vi "Force Measurement.vi"() -> ()   [LabVIEW 2017]
uses:
  <vilib>/Analysis/baseanly.llb/Mean (DBL).vi
  Documents/WT-Control/NU-LabVIEW/Globals/mainWTControl.vi
  <vilib>/Analysis/NI_AALBase.lvlib
panel:
  out "Temp 2":dbl(graph)
  out "Fx":dbl(graph)
  out "Start time":timestamp
  out "concatenated string":string
  in  "Stop Button":bool
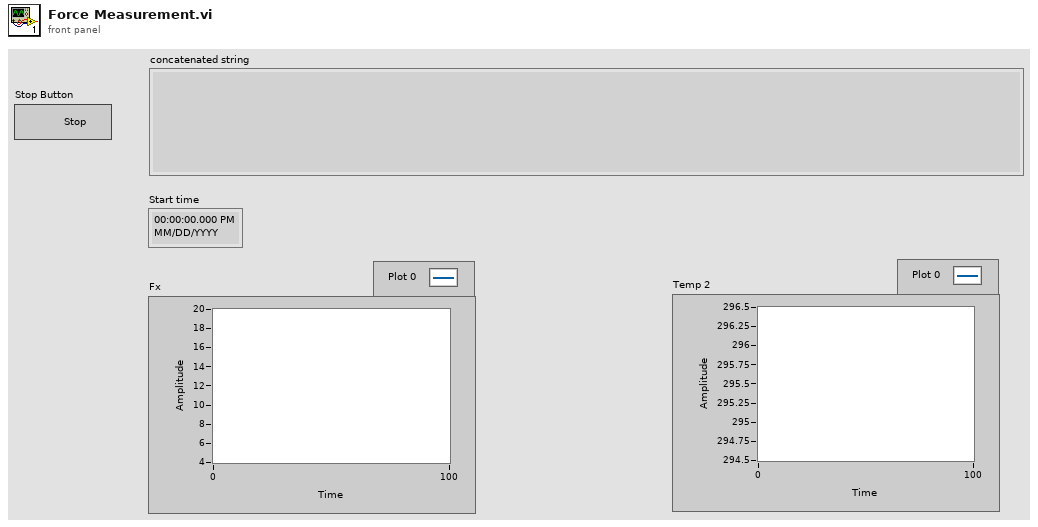
[diagram p1: front panel]
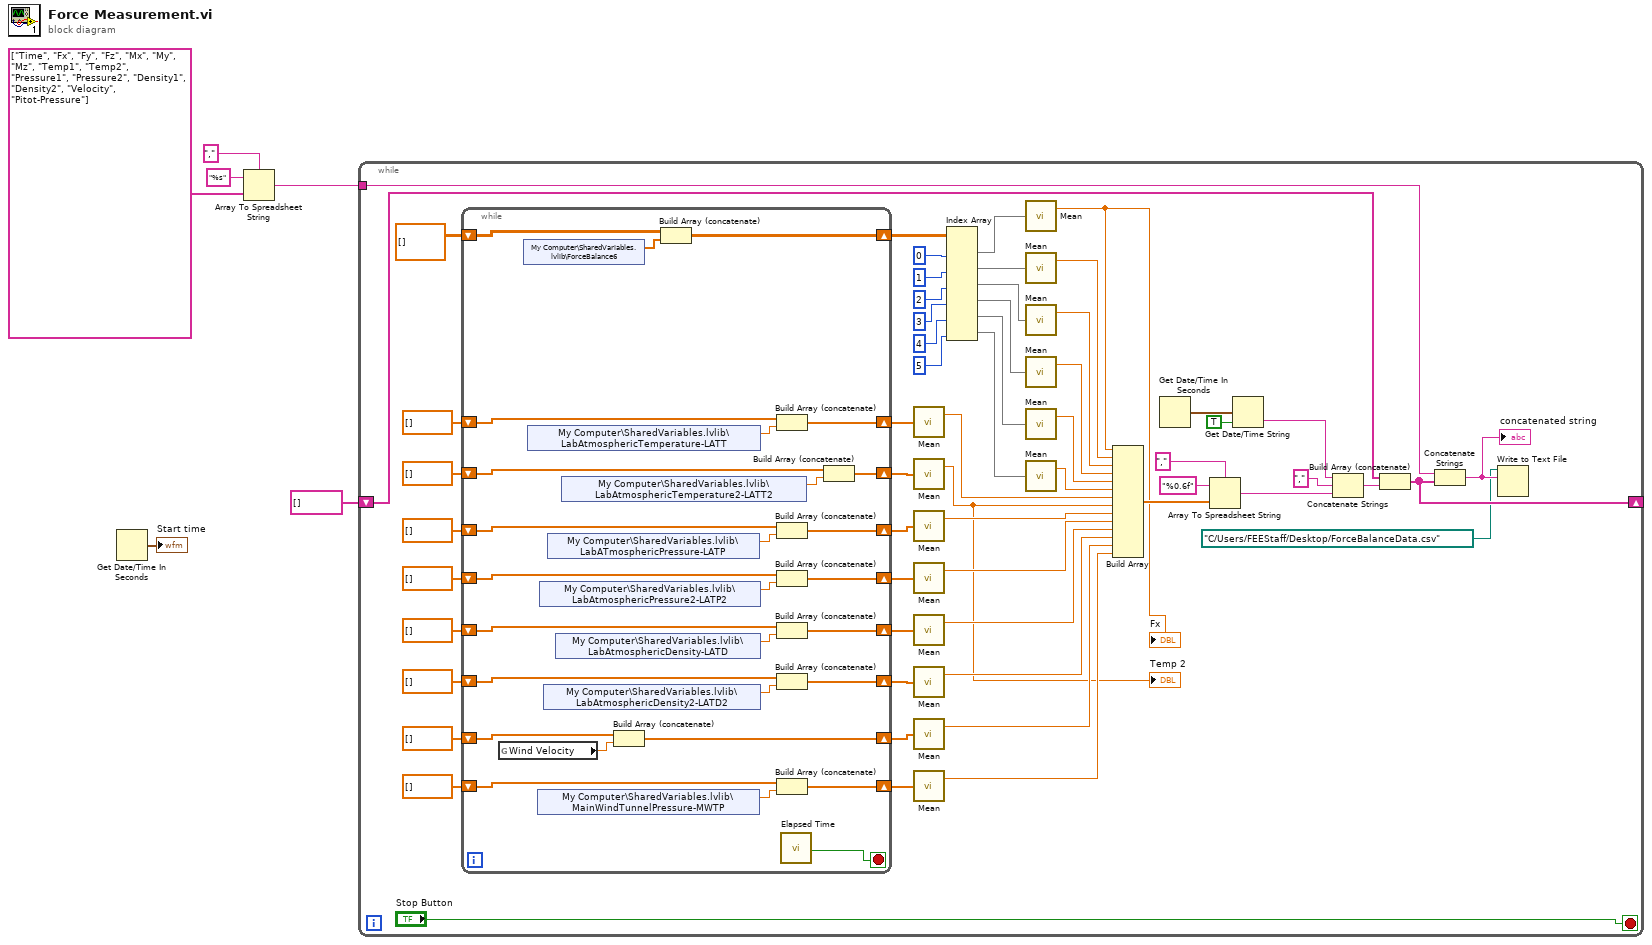
[diagram p0: block diagram]
diagram:
  n1 = Get Date/Time In Seconds() -> (seconds since 1Jan1904=→"Start time":timestamp)
  n2 = Array To Spreadsheet String(delimiter (Tab)=",", array=string[] ["Time", "Fx", "Fy", "Fz", "Mx", "My", "Mz", "Temp1", "Temp2", "Pressure1", "Pressure2", "Density1", "Density2", "Velocity", "Pitot-Pressure"], 3:"%s" ("delimiter (Tab)")) -> (spreadsheet string=w2:string)
  n3 = while {
    shift-right: [w54] -> _
    shift-left: string[] [] -> [w56]
    tunnel: w2 -> [w55]
    stop <- "Stop Button" stop-if-true
    n4 = while {
      shift-right: [w92] -> w52
      shift-left: dbl[][] [] -> [w91]
      shift-right: [w88] -> w38
      shift-left: dbl[] [] -> [w87]
      shift-right: [w73] -> w31
      shift-left: dbl[] [] -> [w66]
      shift-right: [w75] -> w33
      shift-left: dbl[] [] -> [w68]
      shift-right: [w74] -> w32
      shift-left: dbl[] [] -> [w67]
      shift-right: [w76] -> w34
      shift-left: dbl[] [] -> [w69]
      shift-right: [w77] -> w35
      shift-left: dbl[] [] -> [w70]
      shift-right: [w78] -> w36
      shift-left: dbl[] [] -> [w71]
      shift-right: [w85] -> w37
      shift-left: dbl[] [] -> [w72]
      stop <- w90 stop-if-true
      n5 = global read "mainWTControl.vi" "Wind Velocity"() -> (w80:dbl)
      n6 = shared-variable "My Computer\\SharedVariables.lvlib\\ForceBalance6"() -> (w93:dbl[])  [unwired: 1 in, 1 out]
      n7 = shared-variable "My Computer\\SharedVariables.lvlib\\LabAtmosphericTemperature-LATT"() -> (w89:dbl)  [unwired: 1 in, 1 out]
      n8 = shared-variable "My Computer\\SharedVariables.lvlib\\MainWindTunnelPressure-MWTP"() -> (w79:dbl)  [unwired: 1 in, 1 out]
      n9 = shared-variable "My Computer\\SharedVariables.lvlib\\LabAtmosphericPressure2-LATP2"() -> (w83:dbl)  [unwired: 1 in, 1 out]
      n10 = shared-variable "My Computer\\SharedVariables.lvlib\\LabAtmosphericDensity2-LATD2"() -> (w81:dbl)  [unwired: 1 in, 1 out]
      n11 = shared-variable "My Computer\\SharedVariables.lvlib\\LabATmosphericPressure-LATP"() -> (w84:dbl)  [unwired: 1 in, 1 out]
      n12 = shared-variable "My Computer\\SharedVariables.lvlib\\LabAtmosphericDensity-LATD"() -> (w82:dbl)  [unwired: 1 in, 1 out]
      n13 = shared-variable "My Computer\\SharedVariables.lvlib\\LabAtmosphericTemperature2-LATT2"() -> (w86:dbl)  [unwired: 1 in, 1 out]
      n14 = Build Array (concatenate)(w67, w80) -> (w74:dbl[])
      n15 = Build Array (concatenate)(w91, w93) -> (w92:dbl[][])
      n16 = Build Array (concatenate)(w87, w89) -> (w88:dbl[])
      n17 = Build Array (concatenate)(w71, w84) -> (w78:dbl[])
      n18 = Build Array (concatenate)(w70, w83) -> (w77:dbl[])
      n19 = Build Array (concatenate)(w69, w82) -> (w76:dbl[])
      n20 = Build Array (concatenate)(w68, w81) -> (w75:dbl[])
      n21 = Build Array (concatenate)(w66, w79) -> (w73:dbl[])
      n22 = call "Elapsed Time"() -> ("Time has Elapsed"=w90:bool)  [unwired: 12 in, 7 out]
      n23 = Build Array (concatenate)(w72, w86) -> (w85:dbl[])
    }
    n24 = call-poly <vilib>:"Mean.vi"("X"=w38) -> ("mean"=w17:dbl)  [unwired: 1 out]
    n25 = call-poly <vilib>:"Mean.vi"("X"=w37) -> ("mean"=w16:dbl)  [unwired: 1 out]
    "Temp 2" <- w16
    n26 = call-poly <vilib>:"Mean.vi"("X"=w36) -> ("mean"=w25:dbl)  [unwired: 1 out]
    n27 = call-poly <vilib>:"Mean.vi"("X"=w35) -> ("mean"=w24:dbl)  [unwired: 1 out]
    n28 = call-poly <vilib>:"Mean.vi"("X"=w34) -> ("mean"=w23:dbl)  [unwired: 1 out]
    n29 = call-poly <vilib>:"Mean.vi"("X"=w33) -> ("mean"=w22:dbl)  [unwired: 1 out]
    n30 = call-poly <vilib>:"Mean.vi"("X"=w32) -> ("mean"=w21:dbl)  [unwired: 1 out]
    n31 = call-poly <vilib>:"Mean.vi"("X"=w31) -> ("mean"=w20:dbl)  [unwired: 1 out]
    n32 = Index Array(array=w52, index (col) #1=0 ("disabled index (col)"), index (col) #2=1 ("index (col)"), index (col) #3=2 ("index (col)"), index (col) #4=3 ("index (col)"), index (col) #5=4 ("index (col)"), index (col) #6=5 ("index (col)")) -> (element #1=w45:dbl[], element #2=w44:dbl[], element #3=w43:dbl[], element #4=w42:dbl[], element #5=w41:dbl[], element #6=w40:dbl[])  [unwired: 6 in]
    n33 = call-poly <vilib>:"Mean.vi"("X"=w45) -> ("mean"=w7:dbl)  [unwired: 1 out]
    "Fx" <- w7
    n34 = call-poly <vilib>:"Mean.vi"("X"=w44) -> ("mean"=w30:dbl)  [unwired: 1 out]
    n35 = call-poly <vilib>:"Mean.vi"("X"=w43) -> ("mean"=w29:dbl)  [unwired: 1 out]
    n36 = call-poly <vilib>:"Mean.vi"("X"=w42) -> ("mean"=w28:dbl)  [unwired: 1 out]
    n37 = call-poly <vilib>:"Mean.vi"("X"=w41) -> ("mean"=w27:dbl)  [unwired: 1 out]
    n38 = call-poly <vilib>:"Mean.vi"("X"=w40) -> ("mean"=w26:dbl)  [unwired: 1 out]
    n39 = Build Array(w7, w30, w29, w28, w27, w26, w17, w16, w25, w24, w23, w22, w21, w20) -> (w39:dbl[])
    n40 = Get Date/Time In Seconds() -> (seconds since 1Jan1904=w62:timestamp)
    n41 = Array To Spreadsheet String(delimiter (Tab)=",", array=w39, 3:"%0.6f" ("format string")) -> (spreadsheet string=w58:string)
    n42 = Get Date/Time String(seconds (now)=w62, want seconds? (F)=TRUE) -> (time string=w60:string)  [unwired: 1 in, 1 out]
    n43 = Concatenate Strings(w60, "," ("string"), w58) -> (w57:string)
    n44 = Build Array (concatenate)(w56, w57) -> (w54:string[])
    n45 = Concatenate Strings(w55, w54) -> (w19:string)
    "concatenated string" <- w19
    n46 = Write to Text File(file (use dialog)=path "C:/Users/FEEStaff/Desktop/ForceBalanceData.csv", text=w19) -> ()  [unwired: 2 in, 3 out]
  }
